vi "AppleScript Global Data.vi"() -> ()   [LabVIEW 2014]
panel:
  out "Level Reached":bool
  in  "Lift":i16
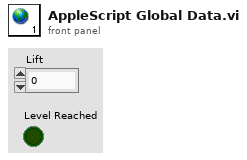
[diagram p1: front panel]
diagram:
